vi "Connect_Arduino&Labview.vi"() -> ()   [LabVIEW 2020]
uses:
  <vilib>/Instr/_visa.llb/VISA Configure Serial Port (Instr).vi
panel:
  out "read buffer":string
  in  "write buffer":string
  in  "stop":bool
  in  "VISA resource name":refnum<visa-resource-name>="COM3"
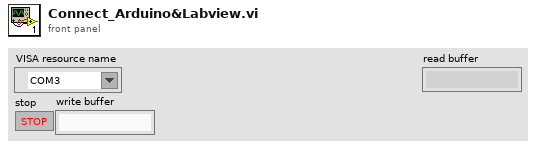
[diagram p1: front panel]
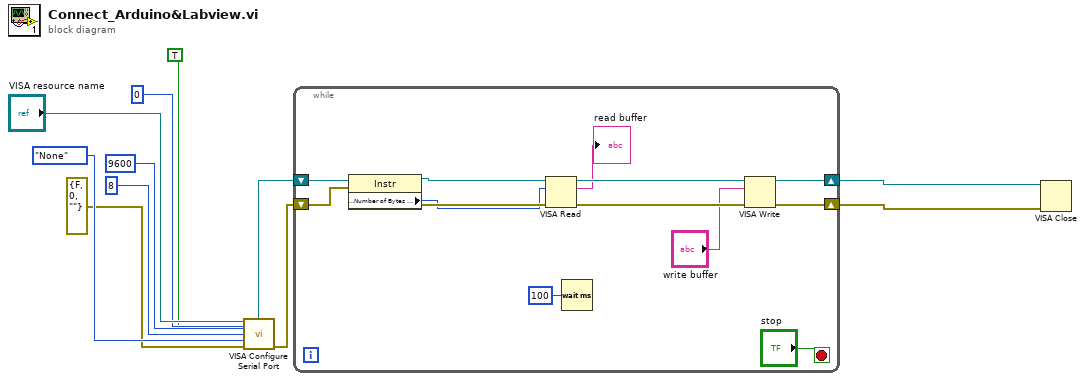
[diagram p0: block diagram]
diagram:
  n1 = call-poly "VISA Configure Serial Port"("VISA resource name"="VISA resource name", "termination char\n(0xA = '\\n' = LF)"=u8 0 ("termination char\n(0xA = '\\n' = LF)"), "Enable Termination\nChar (T)"=TRUE ("Enable Termination\nChar (T)"), "baud rate (9600)"=u32 9600, "data bits (8)"=u16 8, "parity (0:none)"=enum16{"None", "Odd", "Even", "Mark", "Space"}."None", "error in (no error)"=errorcluster {"status"=FALSE, "code"=0, "source"=""}) -> ("VISA resource name out"=w4:refnum<visa-resource-name>, "error out"=w2:errorcluster)  [unwired: 7 in]
  n2 = while {
    shift-right: [w21] -> w3
    shift-left: w4 -> [w24]
    shift-right: [w17] -> w1
    shift-left: w2 -> [w20]
    stop <- "stop" stop-if-true
    n3 = property class="Instr"(reference=w24, error in=w20) -> (reference out=w23:refnum<visa-resource-name>, error out=w19:errorcluster, "Serial Settings:Number of Bytes at Serial Port"=w13:u32)
    n4 = VISA Read(VISA resource name=w23, byte count=w13, error in (no error)=w19) -> (VISA resource name out=w22:refnum<visa-resource-name>, read buffer=→"read buffer":string, error out=w18:errorcluster)  [unwired: 1 out]
    n5 = Wait (ms)(milliseconds to wait=u32 100) -> ()  [unwired: 1 out]
    n6 = VISA Write(VISA resource name=w22, write buffer="write buffer", error in (no error)=w18) -> (VISA resource name out=w21:refnum<visa-resource-name>, error out=w17:errorcluster)  [unwired: 1 out]
  }
  n7 = VISA Close(VISA resource name=w3, error in (no error)=w1) -> ()  [unwired: 1 out]
